vi "Hello.vi"(8 "error in (no error)":errorcluster, 11 "Test Process In":refnum<class "Test Process.lvclass">) -> (0 "error out":errorcluster, 3 "Test Process Out":refnum<class "Test Process.lvclass">)   [LabVIEW 2020, in "Test Process.lvclass"]
uses:
  Test Process.lvclass
  Test Process.lvclass/Test Process.ctl
  <vilib>/Astemes/Triarc Framework/Process/Process.lvclass
  C:/Program Files (x86)/National Instruments/LabVIEW 2020/vi.lib/Astemes/Triarc Framework/Process/Process.lvclass
  C:/Program Files (x86)/National Instruments/LabVIEW 2020/vi.lib/Astemes/Triarc Framework/Base/Base.lvclass
  C:/Program Files (x86)/National Instruments/LabVIEW 2020/vi.lib/Astemes/Triarc Framework/Error Handler Interface/Error Handler Interface.lvclass
  C:/Program Files (x86)/National Instruments/LabVIEW 2020/vi.lib/Astemes/Triarc Framework/Logging/Logging.lvclass
  C:/Users/anton/Documents/GitHub/triarc-debugger/test/Test Process/Test Process.lvclass
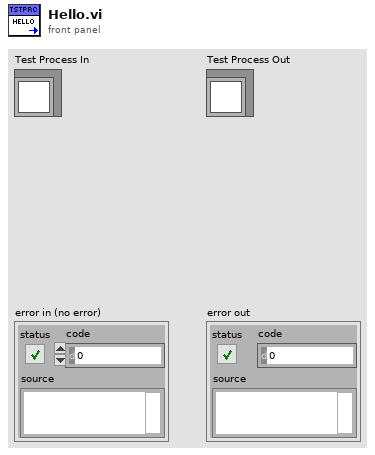
[diagram p1: front panel]
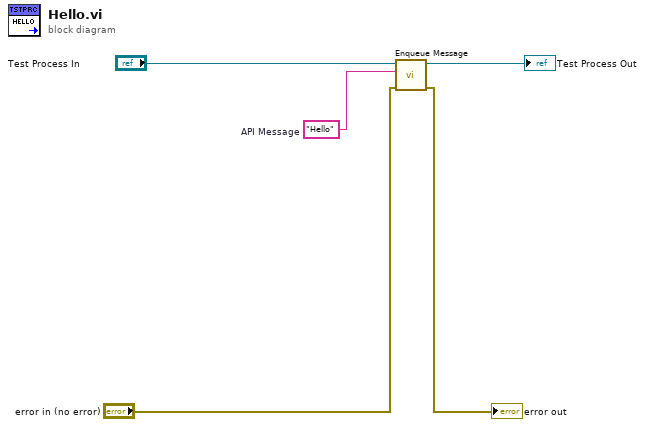
[diagram p0: block diagram]
diagram:
  w2 = "Hello"  # API Message
  n1 = call <vilib>:"Enqueue Message.vi"("error in (no error)"="error in (no error)", "Message"=w2, "Process In"="Test Process In") -> ("error out"=→"error out":errorcluster, "Process Out"=→"Test Process Out":refnum<class "Test Process.lvclass">)  [unwired: 7 in]
